vi "Create Resources.vi"(0 "instance":u8) -> (4 "channel collection builder":refnum<class "Collection Builder.lvclass">, 15 "niUSRP Tx Core":refnum<class "niUSRP Tx Core v1 FPGA.lvclass">)   [LabVIEW 2025, in "niUSRP Tx Core v1 FPGA.lvclass"]
uses:
  niUSRP Tx Core v1 FPGA.lvclass
  <instrlib>/_niInstr/Instruction Framework/v1/FPGA/Collection Builder/Collection Builder.lvclass
  C:/Program Files/NI/LVAddons/niidl/1/instr.lib/_niInstr/Instruction Framework/v1/FPGA/Interfaces/Address Space/Address Space.lvclass
  niUSRP Tx Core v1 FPGA.lvclass/niUSRP Tx Core v1 FPGA.ctl
  <instrlib>/_niInstr/Instruction Framework/v1/FPGA/Helper Classes/Single Address Space Collection/Single Address Space Collection.lvclass
  C:/Program Files/NI/LVAddons/niidl/1/instr.lib/_niInstr/Instruction Framework/v1/FPGA/Interfaces/Address Space Collection/Address Space Collection.lvclass
  <vilib>/rvi/DataTransferAndStorage/Container/Common/niFpgaContainerGetUniqueNameForEmu.vi
  <vilib>/rvi/DataTransferAndStorage/Container/Common/niFpgaContainerSetEmuInfo.vi
  <vilib>/rvi/eio/common/nirviEmuReportErrorAndStop.vi
  <vilib>/rvi/LocalResourceManager/LocalResourceManager.xnode
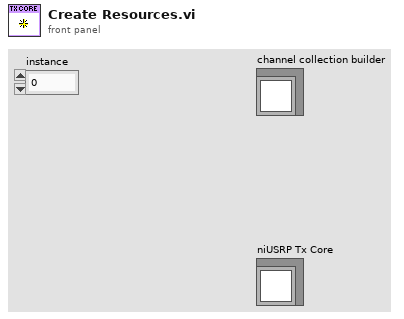
[diagram p1: front panel]
types:
  T1 = typedef "niInstr Address Space Collection Builder v1 FPGA.lvlib/Parent Metadata.ctl" = cluster{"UID":u16, "version":u16, "oldest compatible version":u16}
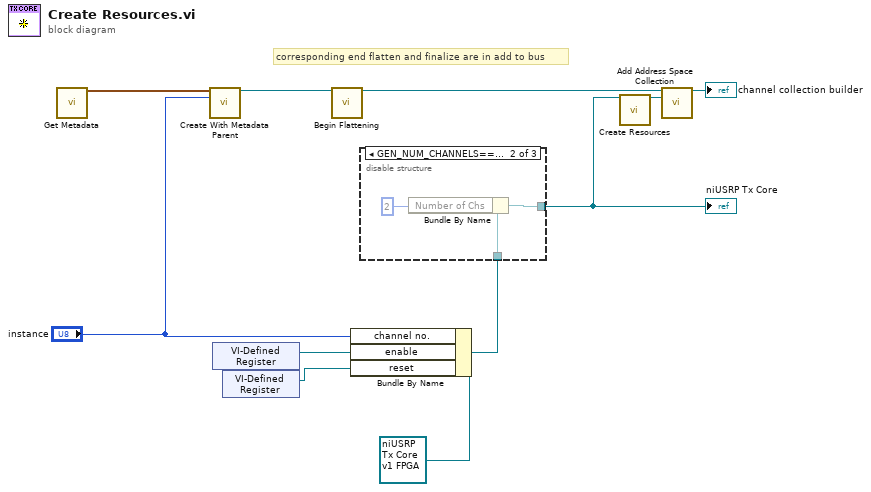
[diagram p0: block diagram]
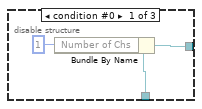
[diagram p2: hidden frame]
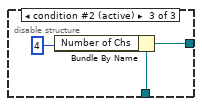
[diagram p3: hidden frame]
diagram:
  # "corresponding end flatten and finalize are in add to bus"
  n1 = call "Get Metadata.vi"() -> ("shared metadata"=w4:T1)  [unwired: 15 in]
  n2 = call <instrlib>:"Create With Metadata Parent.vi"("parent metadata"=w4, "instance (0)"="instance") -> ("collection builder"=w10:refnum<class "Collection Builder.lvclass">)  [unwired: 13 in]
  n3 = xnode "VI-Defined Register"() -> ("Register Out"=w6:refnum<k21>)
  n4 = xnode "VI-Defined Register"() -> ("Register Out"=w5:refnum<k21>)
  n5 = call <instrlib>:"Begin Flattening.vi"("collection builder in"=w10) -> ("collection builder out"=w8:refnum<class "Collection Builder.lvclass">)  [unwired: 14 in]
  n6 = Bundle By Name(cluster=refnum<class "niUSRP Tx Core v1 FPGA.lvclass"> refnum ("niVST Common Reference FPGA.lvclass"), "channel no."="instance", "enable"=w6, "reset"=w5) -> (w3:refnum<class "niUSRP Tx Core v1 FPGA.lvclass">)
  n7 = disable-structure shown="GEN_NUM_CHANNELS==2" {
    disable-tunnel: w3 -> [w14 w17 w18]
    disable-tunnel: [w13 w16 w19] -> w2
    frame condition #0 {
      n8 = Bundle By Name(cluster=w14, "Number of Chs"=u8 1) -> (w13:refnum<class "niUSRP Tx Core v1 FPGA.lvclass">)
    }
    frame condition #1 {
      n9 = Bundle By Name(cluster=w17, "Number of Chs"=u8 2) -> (w16:refnum<class "niUSRP Tx Core v1 FPGA.lvclass">)
    }
    frame condition #2 (active) {
      n10 = Bundle By Name(cluster=w18, "Number of Chs"=u8 4) -> (w19:refnum<class "niUSRP Tx Core v1 FPGA.lvclass">)
    }
  }
  "niUSRP Tx Core" <- w2
  n11 = call <instrlib>:"Create Resources.vi"("address space"=w2) -> ("single address space collection"=w7:refnum<class "Single Address Space Collection.lvclass">)  [unwired: 14 in]
  n12 = call <instrlib>:"Add Address Space Collection.vi"("collection builder in"=w8, "address space collection"=w7) -> ("collection builder out"=→"channel collection builder":refnum<class "Collection Builder.lvclass">)  [unwired: 13 in]
